vi "ConfigInputFeed.vi"(1 "MulticolumnListbox in":refnum<vi>, 3 "ItemNames in":string[][](array[string])) -> (0 "ItemNames out":string[][](array[string]))   [LabVIEW 2018, in "Config.lvlib"]
uses:
  Config.lvlib
panel:
  in  "Replace":bool
  in  "Insert":bool
  in  "Append":bool
  in  "Ring":u8(ring)=1 items=["All", "1", "2", "3", "4", "5", "6", "7", "8"]
  in  "Feed Ratio":dbl=1.0 min=0.05 max=100.0 format="%.2f %"
  # "Feed"
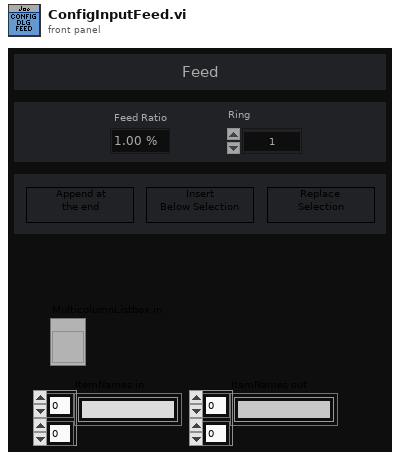
[diagram p1: front panel]
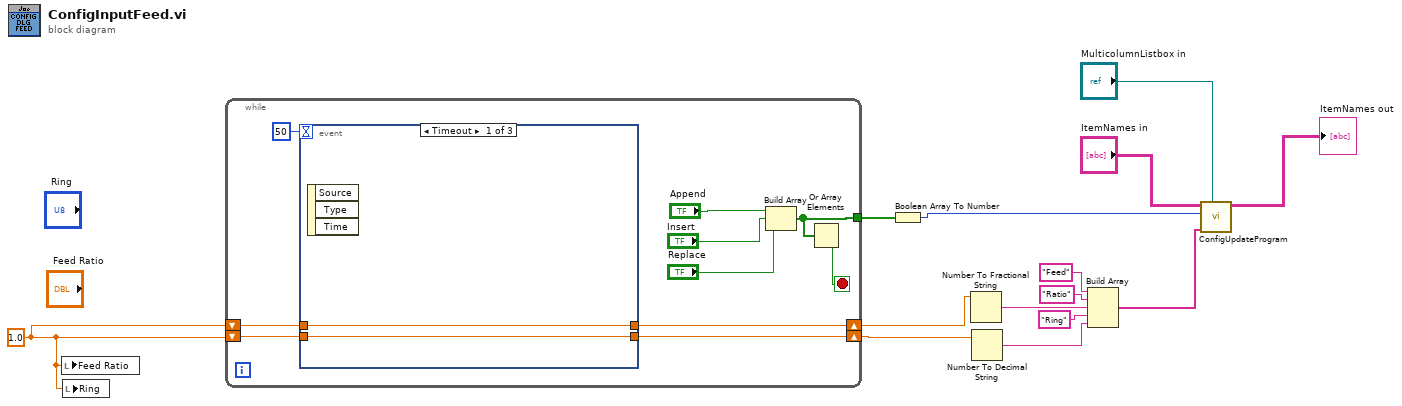
[diagram p0: block diagram]
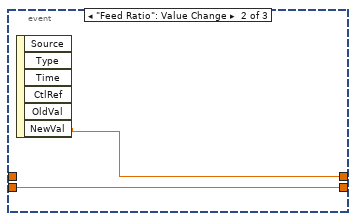
[diagram p2: hidden frame]
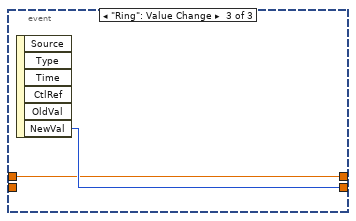
[diagram p3: hidden frame]
diagram:
  w1 = 1.0 ("Mixing Cycles")
  n1 = local write "Feed Ratio"(w1) -> ()
  n2 = local write "Ring"(w1) -> ()
  n3 = while {
    tunnel: [w19] -> w14
    shift-right: [w18] -> w4
    shift-left: w1 -> [w17]
    shift-right: [w16] -> w3
    shift-left: w1 -> [w15]
    stop <- w20 stop-if-true
    n4 = event shown="[0] Timeout" {
      selector: _ -> [_ _ _]
      dyn-events: _ -> [_ _ _]
      timeout: 50 -> [_ _ _]
      tunnel: [w26 w28 w29] -> w18
      tunnel: w17 -> [w26 _ w29]
      tunnel: [w25 w27 w30] -> w16
      tunnel: w15 -> [w25 w27 _]
      event Timeout {
        n5 = event-data() -> ()  [unwired: 1 in, 3 out]
      }
      event "Feed Ratio": Value Change {
        n6 = event-data() -> ("NewVal"=w28:dbl)  [unwired: 1 in, 5 out]
      }
      event "Ring": Value Change {
        n7 = event-data() -> ("NewVal"=w30:u8)  [unwired: 1 in, 5 out]
      }
    }
    n8 = Build Array("Append", "Insert", "Replace") -> (w19:bool[])
    n9 = Or Array Elements(Boolean array=w19) -> (logical OR=w20:bool)
  }
  n10 = Boolean Array To Number(Boolean array=w14) -> (number=w13:u32)
  n11 = Number To Fractional String(number=w4) -> (F-format string=w8:string)  [unwired: 3 in]
  n12 = Number To Decimal String(number=w3) -> (decimal integer string=w6:string)  [unwired: 1 in]
  n13 = Build Array("Feed", "Ratio", w8, "Ring" ("element"), w6) -> (w2:string[])
  n14 = call "ConfigUpdateProgram.vi"("MulticolumnListbox in"="MulticolumnListbox in", "New Element"=w2, "Operation"=w13, "ItemNames in"="ItemNames in") -> ("ItemNames out"=→"ItemNames out":string[][])  [unwired: 7 in]
